vi "Append Heading.vi"(8 "error in (no error)":errorcluster, 9 "Heading Level (-1)":i32=-1, 10 "Heading Text":string, 11 "MS-Word in":refnum<class "MS-Word.lvclass">) -> (0 "error out":errorcluster, 3 "MS-Word out":refnum<class "MS-Word.lvclass">)   [LabVIEW 2017, in "LabVIEW NPOI.lvlib" / "MS-Word.lvclass"]
uses:
  MS-Word.lvclass
  Styles/Title/Title.lvclass
  C:/Users/Neo/Desktop/Dev_Tools_BR/LabVIEW_NPOI/src/Styles/Style/Style.lvclass
  Styles/Heading 1/Heading 1.lvclass
  Styles/Heading 2/Heading 2.lvclass
  Styles/Heading 3/Heading 3.lvclass
  Styles/Style/Style.lvclass
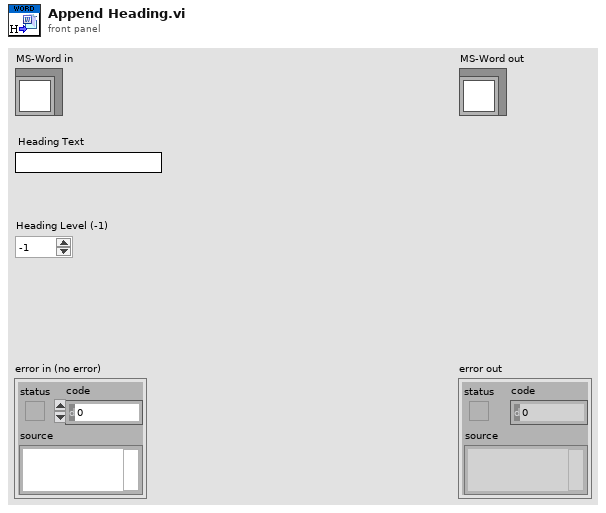
[diagram p1: front panel]
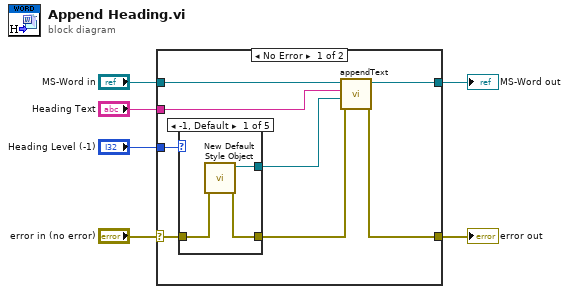
[diagram p0: block diagram]
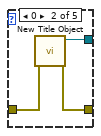
[diagram p2: hidden frame]
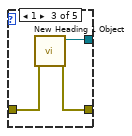
[diagram p3: hidden frame]
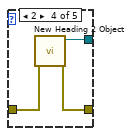
[diagram p4: hidden frame]
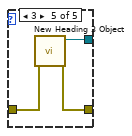
[diagram p5: hidden frame]
diagram:
  n1 = case shown="No Error" "error in (no error)" {
    selector: "error in (no error)" -> [w14 w31]
    tunnel: [w7 w31] -> w5
    tunnel: [w11 w30] -> w3
    tunnel: "MS-Word in" -> [w12 w30]
    tunnel: "Heading Level (-1)" -> [w13 _]
    tunnel: "Heading Text" -> [w10 _]
    frame No Error {
      n2 = case shown="-1, Default" w13 {
        tunnel: w14 -> [w17 w20 w23 w26 w29]
        tunnel: [w16 w19 w22 w25 w28] -> w8
        tunnel: [w15 w18 w21 w24 w27] -> w9
        frame -1, Default {
          n3 = call "New Default Style Object.vi"("error in (no error)"=w17) -> ("error out"=w16:errorcluster, "Style out"=w15:refnum<class "Style.lvclass">)  [unwired: 9 in]
        }
        frame 0 {
          n4 = call "New Title Object.vi"("error in (no error)"=w20) -> ("error out"=w19:errorcluster, "Title out"=w18:refnum<class "Title.lvclass">)  [unwired: 9 in]
        }
        frame 1 {
          n5 = call "New Heading 1 Object.vi"("error in (no error)"=w23) -> ("error out"=w22:errorcluster, "Heading 1 out"=w21:refnum<class "Heading 1.lvclass">)  [unwired: 9 in]
        }
        frame 2 {
          n6 = call "New Heading 2 Object.vi"("error in (no error)"=w26) -> ("error out"=w25:errorcluster, "Heading 2 out"=w24:refnum<class "Heading 2.lvclass">)  [unwired: 9 in]
        }
        frame 3 {
          n7 = call "New Heading 3 Object.vi"("error in (no error)"=w29) -> ("error out"=w28:errorcluster, "Heading 3 out"=w27:refnum<class "Heading 3.lvclass">)  [unwired: 9 in]
        }
      }
      n8 = call-dynamic "appendText.vi"("error in (no error)"=w8, "Style"=w9, "Text"=w10, "MS-Word in"=w12) -> ("error out"=w7:errorcluster, "MS-Word out"=w11:refnum<class "MS-Word.lvclass">)  [unwired: 6 in]
    }
    frame Error {
    }
  }
  "error out" <- w5
  "MS-Word out" <- w3
